vi "Write Mosaic Positions.vi"(11 "path":path=path "C:/Users/BOAS-USER/Documents/Data/0507/human") -> (3 "appended path":path)   [LabVIEW 2018]
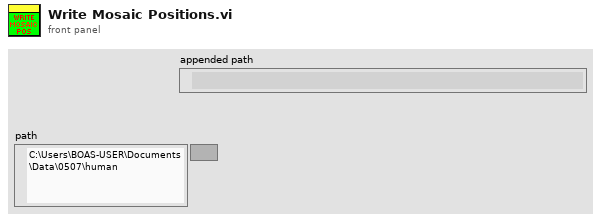
[diagram p1: front panel]
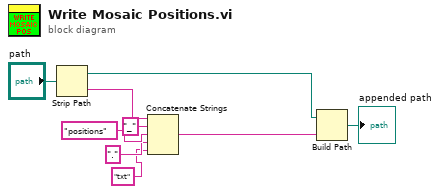
[diagram p0: block diagram]
diagram:
  n1 = Strip Path(path="path") -> (stripped path=w7:path, name=w6:string)
  n2 = Concatenate Strings(w6, "_" ("string"), "positions" ("string"), "." ("string"), "txt" ("string")) -> (w1:string)
  n3 = Build Path(base path=w7, name or relative path=w1) -> (appended path=→"appended path":path)
